vi "Find Average Center.vi"(5 "Position":i32, 7 "Tray Number":i32, 9 "XYZTheta":dbl[](array[numeric]), 10 "Motion.lvclass":refnum<class "Motion.lvclass">) -> (1 "XYZTheta":dbl[](array[numeric]), 2 "Motion Out":refnum<class "Motion.lvclass">)   [LabVIEW 2016, in "Component Tray.lvclass"]
uses:
  Component Tray.lvclass
  Controller/Motion/Motion.lvclass
  Controller/Camera/Edmund Optics/Edmund Optics.lvclass
  Controller/Camera/Camera.lvclass
  C:/Users/HEP Gantry/Documents/GitHub/UCSB-Gantry/V5/Classes/Controller/Camera/Camera.lvclass
  Find Component.ctl
  Controller/Camera/Machine Vision.ctl
panel:
  in  "Machine Vision":T1=enum."Tray Fiducials"
  out "Gantry":dbl[](array[numeric])
  out "Sum":dbl[](array[numeric])
  out "BR XY":dbl[](array[numeric])
  out "TR XY":dbl[](array[numeric])
  out "BL XY":dbl[](array[numeric])
  out "TL XY":dbl[](array[numeric])
  in  "Record Top Right":bool
  in  "Record Bottom Right":bool
  in  "Record Bottom Left":bool
  in  "Record Top Left":bool
  in  "Go to Bottom Right":bool
  in  "Go to Top Right":bool
  in  "Go to Bottom Left":bool
  in  "Go to Top Left":bool
  in  "Joystick":bool
  out "Camera":dbl[](array[numeric])
  in  "Go to Center":bool
  in  "Component":T2
  in  "Stop Program":bool
  out "Image":T3(plugin-control)
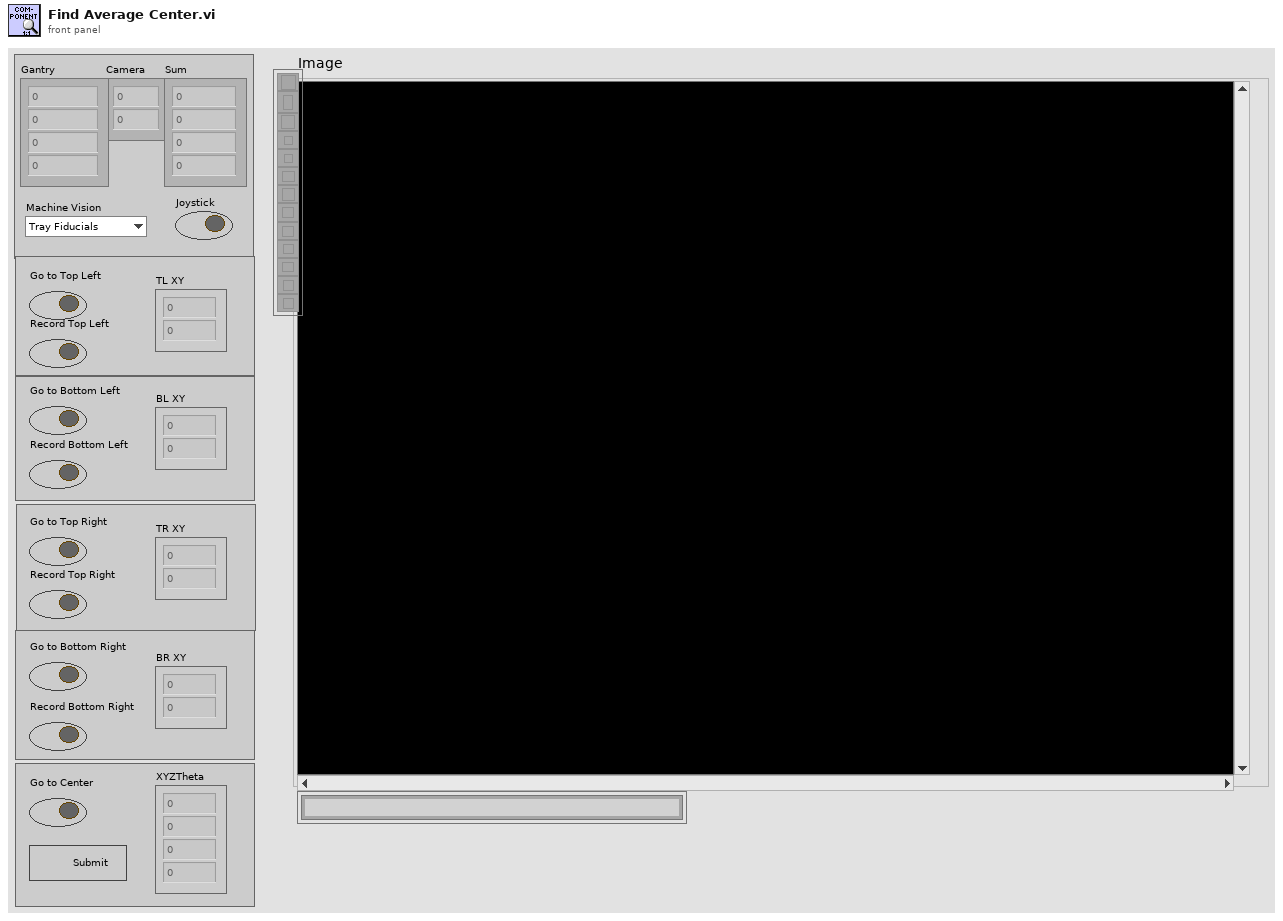
[diagram p1: front panel]
types:
  T1 = typedef "Camera.lvclass/Machine Vision.ctl" = enum16{"None", "Tray Fiducials", "HPK Silicon", "Hexaboard", "Corner (TL, BR)", "Corner (BL, TR)"}
  T2 = typedef "Component Tray.lvclass/Find Component.ctl" = cluster{"New Fiducials":dbl[], "Past Fiducials":dbl[], "XYZTheta":dbl[], "Fiducials Path":path, "Position":i32}
  T3 = typedef "IMAQ Image.ctl" = refnum<image>
  T4 = typedef "File Paths.ctl" = cluster{"Glue Pattern Folder":path, "Carrier Tray Folder":path, "Pick Up Tool Fixture Folder":path, "Components Folder":path, "Bellows Tool Offset.txt":path, "Pick Up Tool Offset.txt":path, "Dispense Tip Offset.txt":path, "Log Files":path}
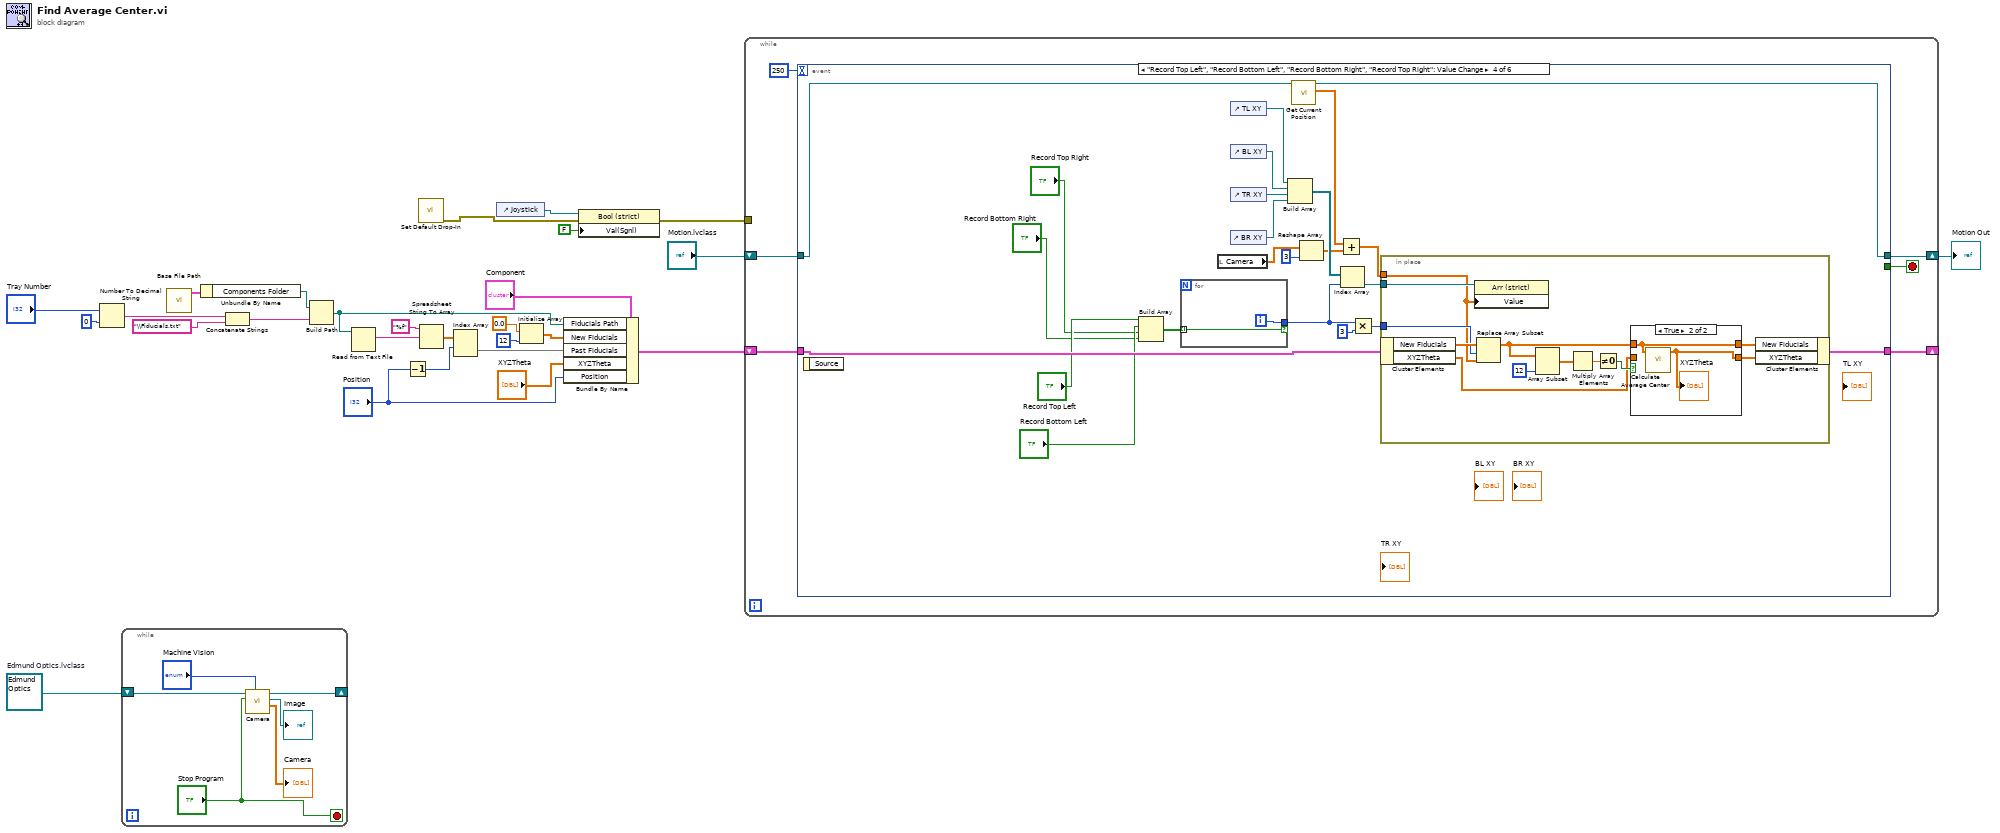
[diagram p0: block diagram]
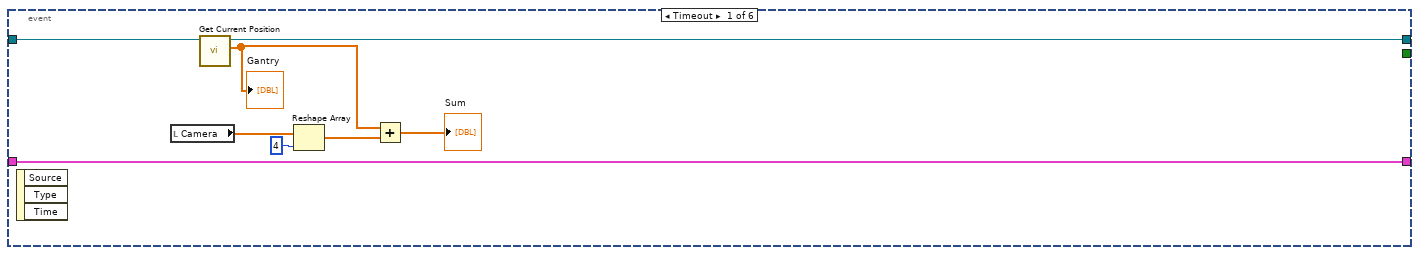
[diagram p2: hidden frame]
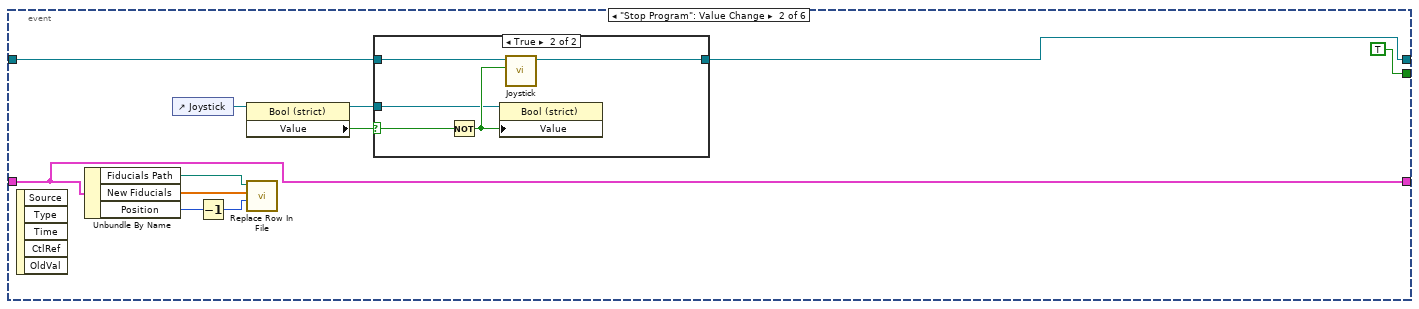
[diagram p3: hidden frame]
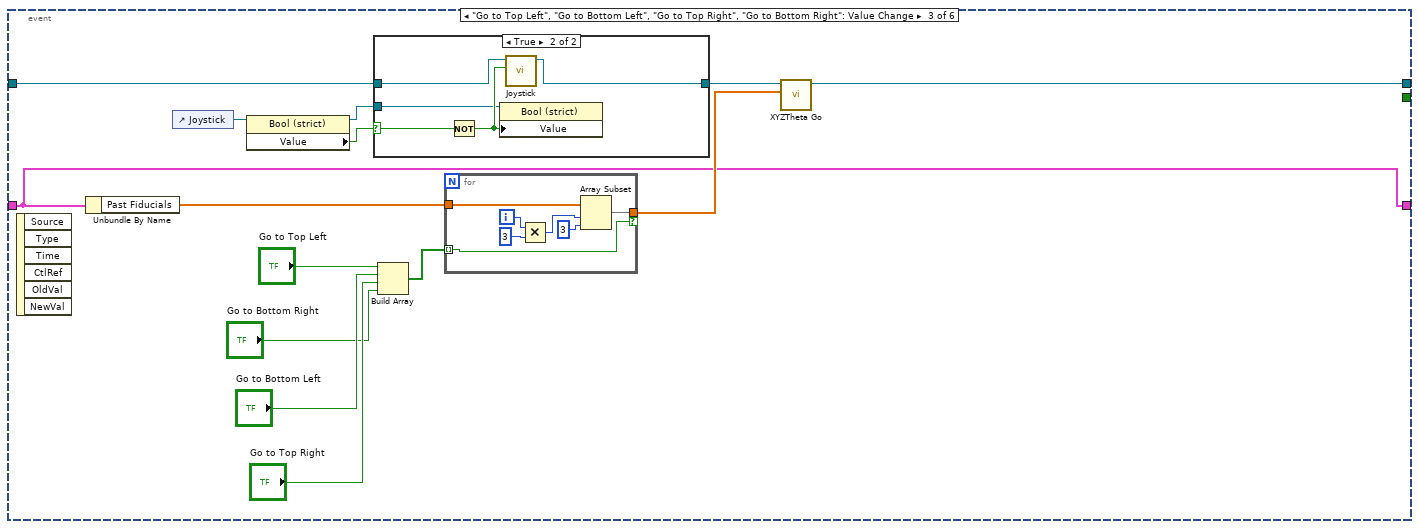
[diagram p5: hidden frame]
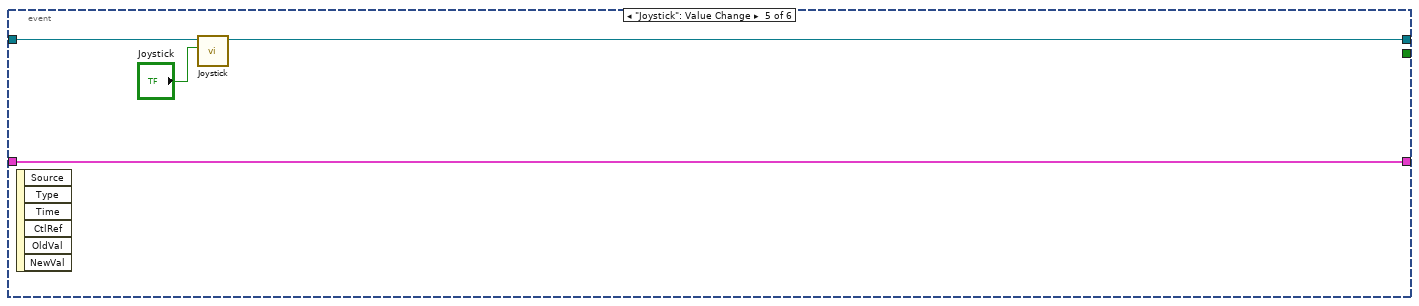
[diagram p8: hidden frame]
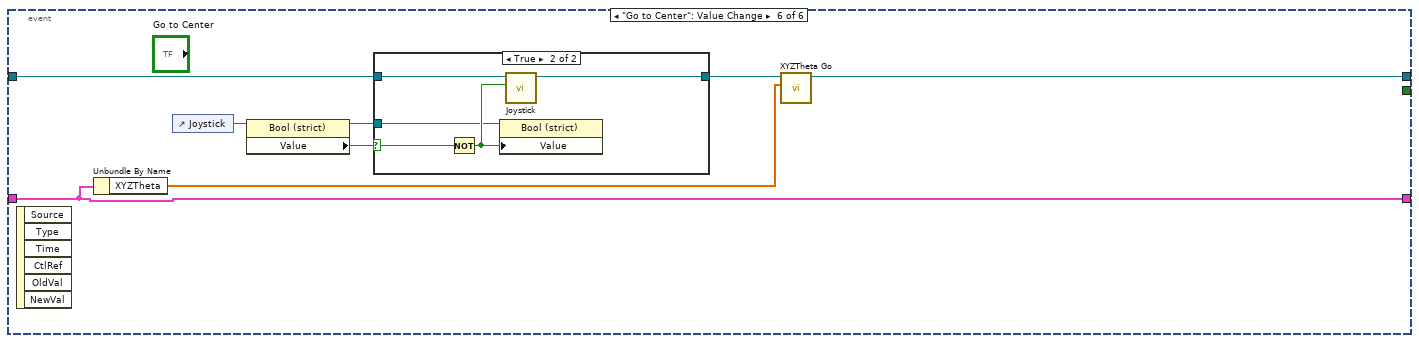
[diagram p9: hidden frame]
diagram:
  w22 = refnum<class "Edmund Optics.lvclass"> refnum  # Edmund Optics.lvclass
  n1 = Number To Decimal String(number="Tray Number", width (-)=i16 0) -> (decimal integer string=w14:string)
  n2 = while {
    shift-right: [w28] -> _
    shift-left: w22 -> [w32]
    stop <- "Stop Program" stop-if-true
    n3 = call "Camera.vi"("Machine Vision"="Machine Vision", "Stop"="Stop Program", "Camera in"=w32) -> ("Camera"=→"Camera":dbl[], "Image"=→"Image":T3, "Camera out"=w28:refnum<class "Edmund Optics.lvclass">)  [unwired: 5 in, 1 out]
  }
  n4 = call "Base File Path.vi"() -> ("Paths Out"=w11:T4)  [unwired: 11 in]
  n5 = Unbundle By Name(w11) -> ("Components Folder"=w13:path)
  n6 = Concatenate Strings(w14, "\\Fiducials.txt" ("string")) -> (w16:string)
  n7 = Build Path(base path=w13, name or relative path=w16) -> (appended path=w5:path)
  n8 = Read from Text File(file (use dialog)=w5) -> (text=w17:string)  [unwired: 3 in, 3 out]
  n9 = Decrement(x="Position") -> (x-1=w2:i32)
  n10 = call "Set Default Drop-In.vi"() -> ("error out"=w1:errorcluster)  [unwired: 11 in]
  n11 = Spreadsheet String To Array(format string="%f", spreadsheet string=w17) -> (array=w19:dbl[][])  [unwired: 2 in]
  n12 = Index Array(array=w19, index (row)=w2) -> (element=w9:dbl[])  [unwired: 1 in]
  n13 = control-ref of="Joystick"() -> (w25:refnum<vi>)
  n14 = Initialize Array(0.0 ("element"), 12 ("dimension size")) -> (w8:dbl[])
  n15 = Bundle By Name(cluster="Component", "Fiducials Path"=w5, "New Fiducials"=w8, "Past Fiducials"=w9, "XYZTheta"="XYZTheta", "Position"="Position") -> (w26:T2)
  n16 = property class="Bool (strict)"(reference=w25, error in=w1, "Val(Sgnl)"=FALSE) -> (error out=w23:errorcluster)  [unwired: 1 out]
  n17 = while {
    shift-right: [w37] -> _
    shift-left: w26 -> [w38]
    tunnel: w23 -> [_]
    shift-right: [w35] -> w20
    shift-left: "Motion.lvclass" -> [w34]
    stop <- w39 stop-if-true
    n18 = event shown="[3] \"Record Top Left\", \"Record Bottom Left\", \"Record Bottom Right\", \"Record Top Right\": Value Change" {
      selector: _ -> [_ _ _ _ _ _]
      dyn-events: _ -> [_ _ _ _ _ _]
      timeout: 250 -> [_ _ _ _ _ _]
      tunnel: [_ TRUE _ _ _ _] -> w39
      tunnel: w38 -> [w44 w52 w71 w114 w135 w142]
      tunnel: [w44 w52 w71 w113 w135 w142] -> w37
      tunnel: w34 -> [w45 w54 w67 w101 w134 w138]
      tunnel: [w43 w53 w70 w100 w133 w143] -> w35
      event Timeout {
        n19 = event-data() -> ()  [unwired: 1 in, 3 out]
        n20 = local read "Camera"() -> (w42:dbl[])
        n21 = call-dynamic "Get Current Position.vi"("Motion in"=w45) -> ("XYZTheta Out"=w46:dbl[], "Motion out"=w43:refnum<class "Motion.lvclass">)  [unwired: 8 in, 1 out]
        "Gantry" <- w46
        n22 = Reshape Array(w42, 4 ("dimension size")) -> (w40:dbl[])
        n23 = Add(x=w46, y=w40) -> (x+y=→"Sum":dbl[])
      }
      event "Stop Program": Value Change {
        n24 = event-data() -> ()  [unwired: 1 in, 5 out]
        n25 = Unbundle By Name(w52) -> ("Fiducials Path"=w50:path, "New Fiducials"=w51:dbl[], "Position"=w49:i32)
        n26 = control-ref of="Joystick"() -> (w55:refnum<vi>)
        n27 = Decrement(x=w49) -> (x-1=w48:i32)
        n28 = property class="Bool (strict)"(reference=w55) -> (reference out=w56:refnum<vi>, "Value"=w57:bool)  [unwired: 1 in, 1 out]
        n29 = call "Replace Row In File.vi"("Index"=w48, "Insert Array"=w51, "Path"=w50) -> ()  [unwired: 8 in, 1 out]
        n30 = case shown="True" w57 {
          selector: w57 -> [_ w64]
          tunnel: w54 -> [w59 w63]
          tunnel: [w59 w62] -> w53
          tunnel: w56 -> [_ w60]
          frame False {
          }
          frame True {
            n31 = Not(x=w64) -> (.not. x?=w61:bool)
            n32 = property class="Bool (strict)"(reference=w60, "Value"=w61) -> ()  [unwired: 1 in, 2 out]
            n33 = call-dynamic "Joystick.vi"("Joystick"=w61, "Motion in"=w63) -> ("Motion out"=w62:refnum<class "Motion.lvclass">)  [unwired: 8 in, 1 out]
          }
        }
      }
      event "Go to Top Left", "Go to Bottom Left", "Go to Top Right", "Go to Bottom Right": Value Change {
        n34 = event-data() -> ()  [unwired: 1 in, 6 out]
        n35 = Unbundle By Name(w71) -> ("Past Fiducials"=w73:dbl[])
        n36 = control-ref of="Joystick"() -> (w65:refnum<vi>)
        n37 = property class="Bool (strict)"(reference=w65) -> (reference out=w68:refnum<vi>, "Value"=w69:bool)  [unwired: 1 in, 1 out]
        n38 = case shown="True" w69 {
          selector: w69 -> [_ w84]
          tunnel: w67 -> [w79 w83]
          tunnel: [w79 w82] -> w66
          tunnel: w68 -> [_ w80]
          frame False {
          }
          frame True {
            n39 = Not(x=w84) -> (.not. x?=w81:bool)
            n40 = property class="Bool (strict)"(reference=w80, "Value"=w81) -> ()  [unwired: 1 in, 2 out]
            n41 = call-dynamic "Joystick.vi"("Joystick"=w81, "Motion in"=w83) -> ("Motion out"=w82:refnum<class "Motion.lvclass">)  [unwired: 8 in, 1 out]
          }
        }
        n42 = Build Array("Go to Top Left", "Go to Bottom Left", "Go to Top Right", "Go to Bottom Right") -> (w74:bool[])
        n43 = for {
          tunnel: w74 -> [w91] mode=indexing
          tunnel: w73 -> [w90]
          tunnel: [w85] -> w72 if=w91
          i -> [w88]
          n44 = Multiply(x=w88, y=3) -> (x*y=w86:i32)
          n45 = Array Subset(array=w90, index=w86, length=3) -> (w85:dbl[])
        }
        n46 = call "XYZTheta Go.vi"("XYZTheta In"=w72, "Motion in"=w66) -> ("Motion out"=w70:refnum<class "Motion.lvclass">)  [unwired: 7 in, 2 out]
      }
      event "Record Top Left", "Record Bottom Left", "Record Bottom Right", "Record Top Right": Value Change {
        n47 = event-data() -> ()  [unwired: 1 in, 1 out]
        n48 = Build Array("Record Top Left", "Record Bottom Left", "Record Top Right", "Record Bottom Right") -> (w108:bool[])
        n49 = for {
          tunnel: w108 -> [w115] mode=indexing
          tunnel: [w116] -> w97 if=w115
          i -> [w116]
        }
        n50 = local read "Camera"() -> (w94:dbl[])
        n51 = control-ref of="TL XY"() -> (w107:refnum<vi>)
        n52 = control-ref of="BL XY"() -> (w106:refnum<vi>)
        n53 = control-ref of="TR XY"() -> (w105:refnum<vi>)
        n54 = control-ref of="BR XY"() -> (w104:refnum<vi>)
        n55 = Build Array(w107, w106, w105, w104) -> (w103:refnum<vi>[])
        n56 = call-dynamic "Get Current Position.vi"("Motion in"=w101) -> ("XYZTheta Out"=w99:dbl[], "Motion out"=w100:refnum<class "Motion.lvclass">)  [unwired: 8 in, 1 out]
        n57 = Reshape Array(w94, 3 ("dimension size")) -> (w93:dbl[])
        n58 = Add(x=w99, y=w93) -> (x+y=w92:dbl[])
        n59 = Index Array(array=w103, index=w97) -> (element=w102:refnum<vi>)
        n60 = Multiply(x=w97, y=3) -> (x*y=w95:i32)
        n61 = in-place {
          in-place-border: w95 -> [w126]
          in-place-border: w102 -> [w123]
          in-place-border: w92 -> [w121]
          n62 = in-place-cluster #1(w114) -> ("New Fiducials"=w127:dbl[], "XYZTheta"=w122:dbl[])
          n63 = property class="Arr (strict)"(reference=w123, "Value"=w121) -> ()  [unwired: 1 in, 2 out]
          n64 = Replace Array Subset(array=w127, new element=w121, index=w126) -> (w120:dbl[])
          n65 = Array Subset(array=w120, length=12) -> (w118:dbl[])  [unwired: 1 in]
          n66 = Multiply Array Elements(1:w118) -> (0:w117:dbl)
          n67 = Not Equal To 0?(x=w117) -> (x != 0?=w124:bool)
          n68 = case shown="True" w124 {
            tunnel: [w129 w131] -> w128
            tunnel: w120 -> [w130 w132]
            tunnel: [w130 w132] -> w125
            tunnel: w122 -> [w129 _]
            frame False {
            }
            frame True {
              n69 = call "Calculate Average Center.vi"("Gantry Fiducials"=w132) -> ("XYZTheta"=w131:dbl[])  [unwired: 10 in]
              "XYZTheta" <- w131
            }
          }
          n70 = in-place-cluster #1("New Fiducials"=w125, "XYZTheta"=w128) -> (w113:T2)
        }
      }
      event "Joystick": Value Change {
        n71 = event-data() -> ()  [unwired: 1 in, 6 out]
        n72 = call-dynamic "Joystick.vi"("Joystick"="Joystick", "Motion in"=w134) -> ("Motion out"=w133:refnum<class "Motion.lvclass">)  [unwired: 8 in, 1 out]
      }
      event "Go to Center": Value Change {
        n73 = event-data() -> ()  [unwired: 1 in, 6 out]
        n74 = Unbundle By Name(w142) -> ("XYZTheta"=w144:dbl[])
        n75 = control-ref of="Joystick"() -> (w139:refnum<vi>)
        n76 = property class="Bool (strict)"(reference=w139) -> (reference out=w140:refnum<vi>, "Value"=w141:bool)  [unwired: 1 in, 1 out]
        n77 = case shown="True" w141 {
          selector: w141 -> [_ w150]
          tunnel: w138 -> [w145 w149]
          tunnel: [w145 w148] -> w137
          tunnel: w140 -> [_ w146]
          frame False {
          }
          frame True {
            n78 = Not(x=w150) -> (.not. x?=w147:bool)
            n79 = property class="Bool (strict)"(reference=w146, "Value"=w147) -> ()  [unwired: 1 in, 2 out]
            n80 = call-dynamic "Joystick.vi"("Joystick"=w147, "Motion in"=w149) -> ("Motion out"=w148:refnum<class "Motion.lvclass">)  [unwired: 8 in, 1 out]
          }
        }
        n81 = call "XYZTheta Go.vi"("XYZTheta In"=w144, "Motion in"=w137) -> ("Motion out"=w143:refnum<class "Motion.lvclass">)  [unwired: 7 in, 2 out]
      }
    }
  }
  "Motion Out" <- w20
